vi "getrMethods.vi"(0 "reference":refnum<class "InterfaceNode.lvclass">, 5 "error in (no error)":errorcluster) -> (14 "reference out":refnum<class "InterfaceNode.lvclass">, 15 "methods":refnum<class "MultiLineString.lvclass">, 19 "error out":errorcluster)   [LabVIEW 2020, in "InterfaceNode.lvclass"]
doc: "public MultiLineString getMethods()"
uses:
  <resource>/Framework/Providers/Open_GDS/UML/InterfaceNode_class/InterfaceNode.lvclass
  C:/Program Files (x86)/National Instruments/LabVIEW 2020/resource/Framework/Providers/Open_GDS/UML/ClassNode_class/ClassNode.lvclass
  <resource>/Framework/Providers/Open_GDS/UML/MultiLineString_class/MultiLineString.lvclass
  <resource>/Framework/Providers/Open_GDS/UML/ClassNode_class/ClassNode.lvclass
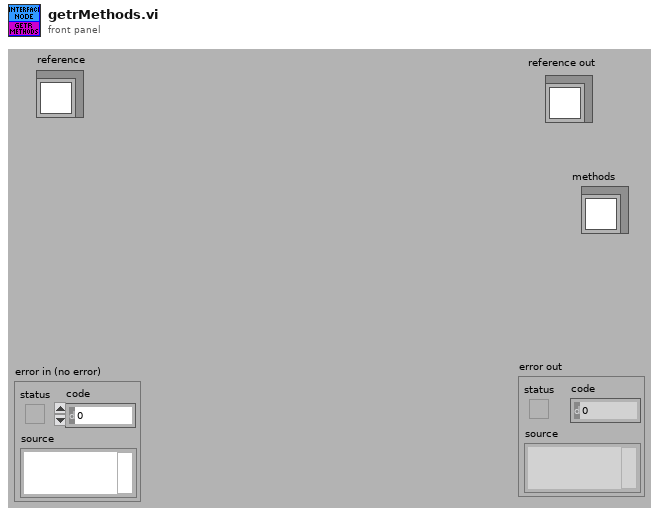
[diagram p1: front panel]
types:
  T1 = typedef "ClassNode.lvclass/ObjectAttributes.ctl" = cluster{"midHeight":dbl, "botHeight":dbl, "name":refnum<class "MultiLineString.lvclass">, "attributes":refnum<class "MultiLineString.lvclass">, "methods":refnum<class "MultiLineString.lvclass">, "DEFAULT_COMPARTMENT_HEIGHT":i32, "DEFAULT_WIDTH":i32, "DEFAULT_HEIGHT":i32, "showMethods":bool, "showAttributes":bool, "ClassPath":path}
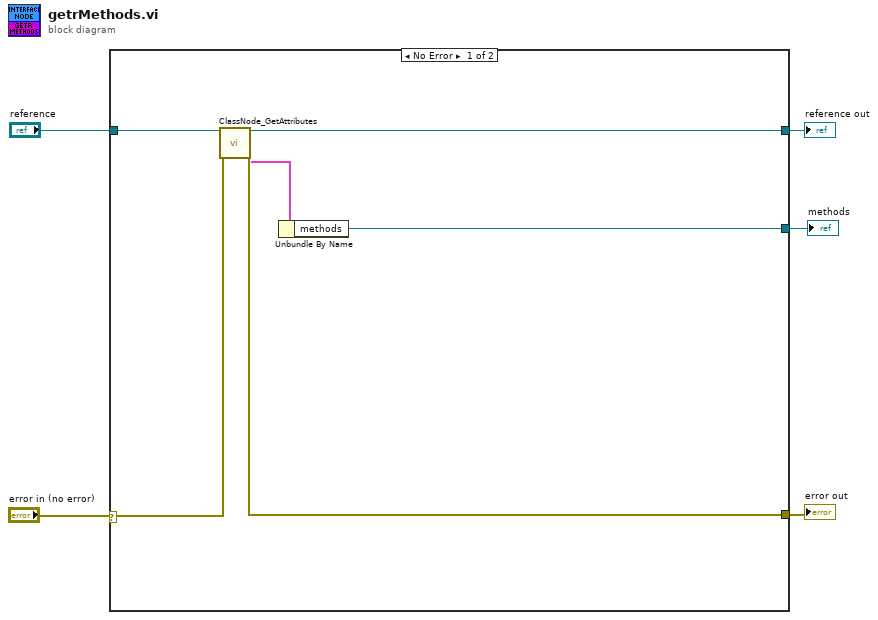
[diagram p0: block diagram]
diagram:
  n1 = case shown="No Error" "error in (no error)" {
    selector: "error in (no error)" -> [w8 w12]
    tunnel: "reference" -> [w11 w13]
    tunnel: [w10 w12] -> w4
    tunnel: [w9 w13] -> w3
    tunnel: [w7 _] -> w1
    frame No Error {
      n2 = call <resource>:"ClassNode_GetAttributes.vi"("reference in"=w11, "error in (no error)"=w8) -> ("reference out"=w9:refnum<class "InterfaceNode.lvclass">, "Data"=w6:T1, "error out"=w10:errorcluster)  [unwired: 14 in, 1 out]
      n3 = Unbundle By Name(w6) -> ("methods"=w7:refnum<class "MultiLineString.lvclass">)
    }
    frame Error {
    }
  }
  "reference out" <- w3
  "error out" <- w4
  "methods" <- w1
